vi "create event queues.vi"(11 "sizes":i32[](array[numeric])) -> (3 "event queue":T1)   [LabVIEW 2013, in "data bus events.lvlib"]
uses:
  data bus events.lvlib
  event queue.ctl
  event queue element.ctl
  event.ctl
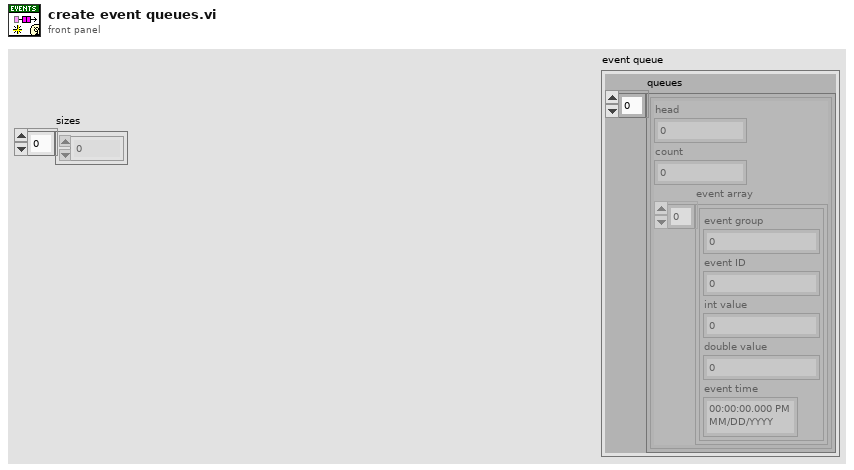
[diagram p1: front panel]
types:
  T1 = typedef "data bus events.lvlib/event queue.ctl" = cluster{"queues":T2[]}
  T2 = typedef "data bus events.lvlib/event queue element.ctl" = cluster{"head":i32, "count":i32, "event array":T3[]}
  T3 = typedef "data bus events.lvlib/event.ctl" = cluster{"event group":i64, "event ID":i64, "int value":i64, "double value":dbl, "event time":timestamp}
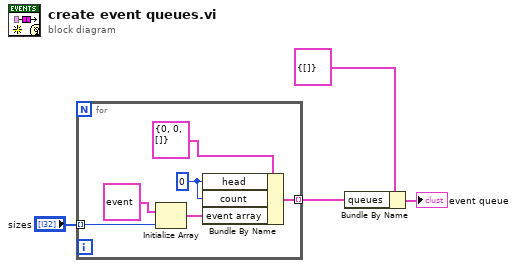
[diagram p0: block diagram]
diagram:
  n1 = for {
    tunnel: [w8] -> w2 mode=indexing
    tunnel: "sizes" -> [w5] mode=indexing
    w9 = 0 ("count")
    n2 = Initialize Array(T3 {"event group"=0, "event ID"=0, "int value"=0, "double value"=0.0, "event time"=timestamp(0 s since 1904-01-01)} ("event"), w5) -> (w6:T3[])
    n3 = Bundle By Name(cluster=T2 {"head"=0, "count"=0, "event array"=[]} ("event queue element"), "head"=w9, "count"=w9, "event array"=w6) -> (w8:T2)
  }
  n4 = Bundle By Name(cluster=T1 {"queues"=[]} ("event queue"), "queues"=w2) -> (→"event queue":T1)
